vi "Request Control Update.vi"(8 "error in (no error)":errorcluster, 11 "Operator in":refnum<class "Operator.lvclass">) -> (0 "error out":errorcluster, 3 "Operator out":refnum<class "Operator.lvclass">)   [LabVIEW 2014, in "Operator.lvlib" / "Operator.lvclass"]
uses:
  Operator.lvclass
  Operator.lvclass/Operator.ctl
  Operator Messages/Get Operator Joystick State Msg/Get Operator Joystick State Msg.lvclass
  <vilib>/ActorFramework/Actor/Actor.lvclass/Actor.ctl
  <vilib>/ActorFramework/Message Enqueuer/Message Enqueuer.lvclass/Message Enqueuer.ctl
  Joystick/Joystick Messages/Request Joystick State Msg/Request Joystick State Msg.lvclass/Request Joystick State Msg.ctl
  <vilib>/ActorFramework/Message Enqueuer/Init from Existing Queue.vi
  <vilib>/ActorFramework/Message Enqueuer/Enqueue.vi
  <vilib>/ActorFramework/Message Priority Queue/Priority Enqueue.vi
  <vilib>/ActorFramework/Message Enqueuer/Message Enqueuer.lvclass
  Joystick/Joystick Messages/Request Joystick State Msg/Request Joystick State Msg.lvclass
  <vilib>/ActorFramework/Actor/Actor.lvclass
  Robot Actor Framework/Utilities/Utilities.lvlib
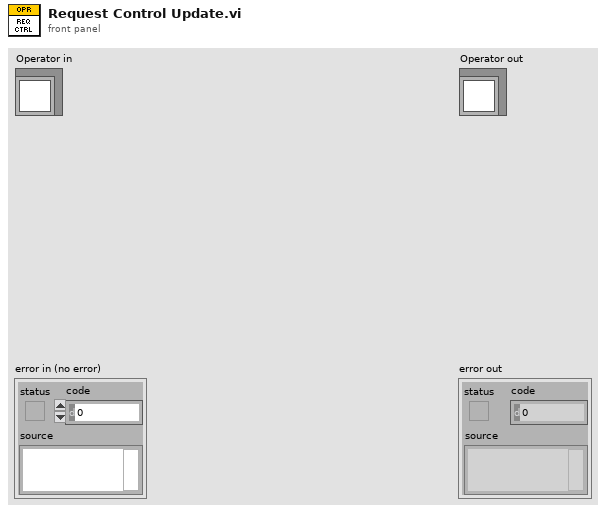
[diagram p1: front panel]
types:
  T1 = enum16{"Critical", "Error", "Warning", "Informational", "Debug"}
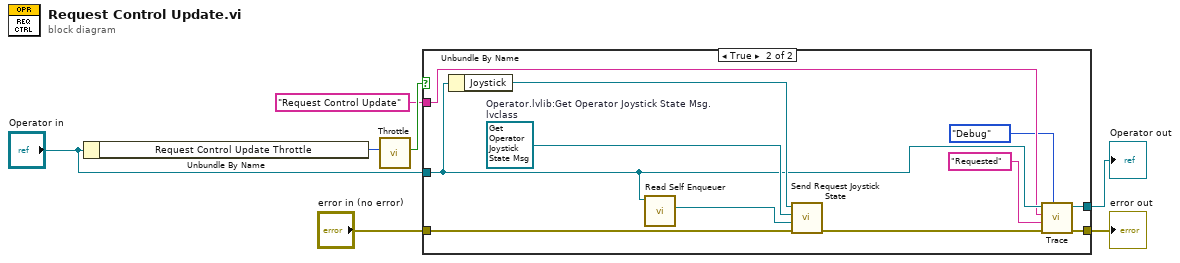
[diagram p0: block diagram]
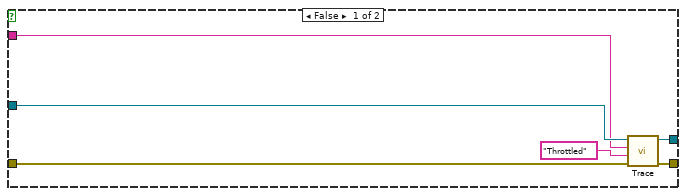
[diagram p2: hidden frame]
diagram:
  n1 = Unbundle By Name("Operator in") -> ("Request Control Update Throttle"=w1:u32)
  n2 = call "Throttle.vi"("Throttle (ms)"=w1) -> ("Past Throttle"=w4:bool)  [unwired: 10 in]
  n3 = case shown="True" w4 {
    tunnel: "error in (no error)" -> [w13 w21]
    tunnel: [w12 w19] -> w6
    tunnel: "Operator in" -> [w11 w18]
    tunnel: [w10 w17] -> w5
    tunnel: "Request Control Update" ("System Action") -> [w9 w15]
    frame False {
      n4 = call-dynamic "Trace.vi"("error in (no error)"=w13, "System Message"="Throttled", "System Action"=w9, "System Actor in"=w11) -> ("error out"=w12:errorcluster, "System Actor out"=w10:refnum<class "Operator.lvclass">)  [unwired: 6 in]
    }
    frame True {
      w23 = refnum<class "Get Operator Joystick State Msg.lvclass"> refnum  # Operator.lvlib:Get Operator Joystick State Msg.lvclass
      n5 = Unbundle By Name(w18) -> ("Joystick"=w24:refnum<class "Message Enqueuer.lvclass">)
      n6 = call <vilib>:"Read Self Enqueuer.vi"("Actor"=w18) -> ("Self Enqueuer"=w22:refnum<class "Message Enqueuer.lvclass">)  [unwired: 10 in]
      n7 = call "Send Request Joystick State.vi"("error in (no error)"=w21, "Caller Enqueuer"=w22, "Joystick State Msg"=w23, "Message Enqueuer"=w24) -> ("error out"=w20:errorcluster)  [unwired: 6 in, 1 out]
      n8 = call-dynamic "Trace.vi"("Trace Level"=T1."Debug", "error in (no error)"=w20, "System Message"="Requested", "System Action"=w15, "System Actor in"=w18) -> ("error out"=w19:errorcluster, "System Actor out"=w17:refnum<class "Operator.lvclass">)  [unwired: 5 in]
    }
  }
  "error out" <- w6
  "Operator out" <- w5
